vi "Apply-threshold-filter.vi"(7 "Threshold only 2nd camera image?":bool, 8 "error in":errorcluster, 9 "Corrected":T1[](array[typedef]), 11 "Noise treshold":sgl) -> (0 "error IO":errorcluster)   [LabVIEW 2013, in "CameraVision.lvlib" / "CV-Correction.lvclass"]
uses:
  CV-Correction.lvclass
  <vilib>/vision/Image Controls.llb/IMAQ Image.ctl
  <vilib>/vision/NI_Vision_Development_Module.lvlib
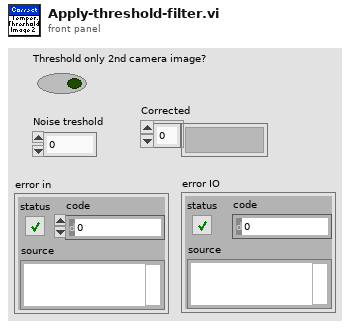
[diagram p1: front panel]
types:
  T1 = typedef "IMAQ Image.ctl" = refnum<image>
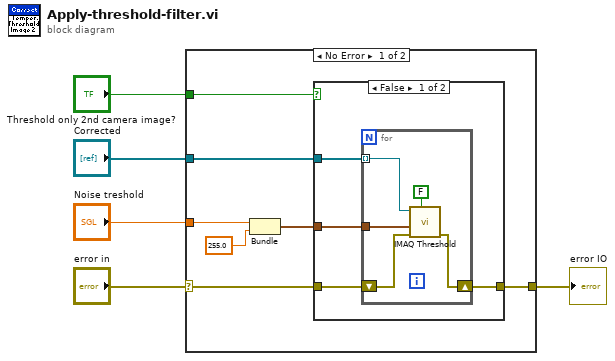
[diagram p0: block diagram]
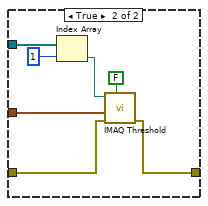
[diagram p2: hidden frame]
diagram:
  n1 = case shown="No Error" "error in" {
    selector: "error in" -> [w9 w29]
    tunnel: [w12 w29] -> w5
    tunnel: "Noise treshold" -> [w8 _]
    tunnel: "Corrected" -> [w7 _]
    tunnel: "Threshold only 2nd camera image?" -> [w6 _]
    frame No Error {
      n2 = Bundle("Noise treshold"=w8, sgl 255.0) -> (w10:cluster{"Noise treshold":sgl, sgl})  [unwired: 1 in]
      n3 = case shown="False" w6 {
        tunnel: [w13 w27] -> w12
        tunnel: w10 -> [w16 w24]
        tunnel: w9 -> [w14 w23]
        tunnel: w7 -> [w15 w22]
        frame False {
          n4 = for {
            tunnel: w16 -> [w20]
            tunnel: w15 -> [w19] mode=indexing
            shift-right: [w17] -> w13
            shift-left: w14 -> [w18]
            n5 = call "IMAQ Threshold"("Keep/Replace Value (Replace)"=FALSE, "error in (no error)"=w18, "Range"=w20, "Image Src"=w19) -> ("error out"=w17:errorcluster)  [unwired: 6 in, 1 out]
          }
        }
        frame True {
          n6 = Index Array(array=w22, index=1) -> (element=w26:T1)
          n7 = call "IMAQ Threshold"("Keep/Replace Value (Replace)"=FALSE, "error in (no error)"=w23, "Range"=w24, "Image Src"=w26) -> ("error out"=w27:errorcluster)  [unwired: 6 in, 1 out]
        }
      }
    }
    frame Error {
    }
  }
  "error IO" <- w5
